vi "ScanDelay_FTIR_GetSpectrum_Aligning_Testing.vi"(0 "Cancel? External":refnum<vi>, 1 "% averaged (external)":refnum<vi>, 2 "Binned interferogram (external)":refnum<vi>, 3 "Python refnum in":refnum<k35>, 5 "Refresh alignment":bool=TRUE, 7 "Acquisition cycle (external)":refnum<vi>, 9 "Delay calibration\n          factor":dbl=2.403, 10 "Python error in":errorcluster, 11 "Subtract\ndelay (ps)":dbl, 12 "Acquisitions per interferogram":i32=20, 13 "Time per\nacquisition (s)":dbl=0.31, 14 "Sampling rate":dbl=250000.0, 15 "Extract envelope":bool=TRUE) -> (4 "Output spectrum":dbl[][](array[numeric]), 6 "Python error out":errorcluster)   [LabVIEW 2021]
uses:
  Control_GetSpectrum_Aligning.ctl
  <vilib>/DAQmx/read.llb/DAQmx Read (Analog 2D DBL NChan NSamp).vi
  <vilib>/DAQmx/miscellaneous.llb/DAQmx Fill In Error Info.vi
panel:
  out "Time per\nloop1 (ms)":dbl=333.0
  out "DAQmx error":errorcluster={"status"=FALSE, "code"=200012, "source"="DAQmx Control Task.vi:3900001"}
  out "Time per\nloop2 (ms)":dbl
  in  "Save interferograms\n(interferograms.txt)":bool
  in  "Alignment order":i32=1
  out "Own python session":bool=TRUE
  out "Refnum errors":errorcluster={"status"=TRUE, "code"=1055, "source"="Property Node in ScanDelay_FTIR_GetSpectrum_Aligning_Testing.vi"}
  out "Spectrum (amplitude)":cluster{dbl[], dbl[]}[](graph)
  out "Spectrum (phase)":cluster{dbl[], dbl[]}(graph)
  out "Interferogram (aligned)":cluster{dbl, dbl}[](graph)
  out "Acquisition cycle":dbl[][](graph)
  in  "Halt acquisition":bool
  out "Python module path":path=path "C:/Users/mnopl/Desktop/Software/LabVIEW/ScanDelay/scandelay.py"
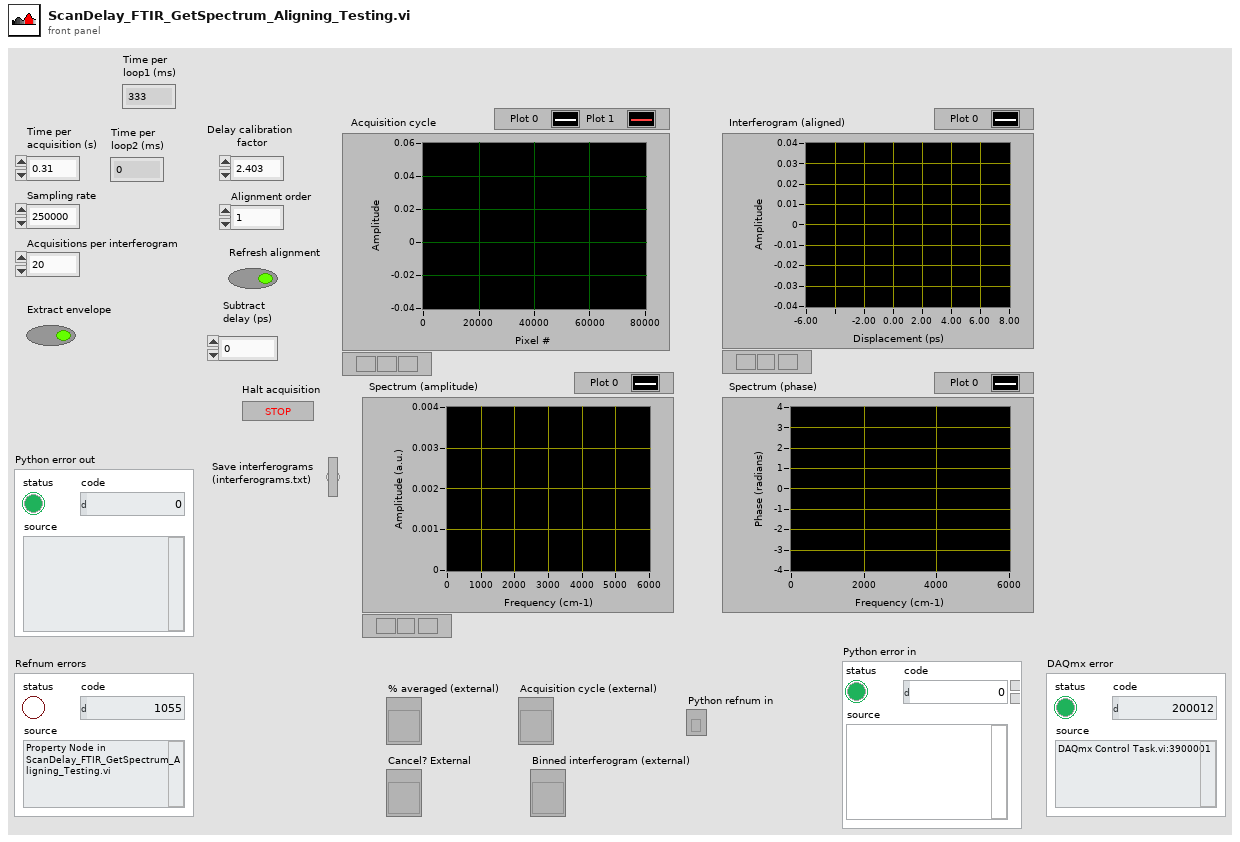
[diagram p1: front panel]
types:
  T1 = typedef "Control_GetSpectrum_Aligning.ctl" = enum16{"Acquire Interferograms", "Prepare DAQ task", "Align Interferograms", "Compute Spectrum", "Done"}
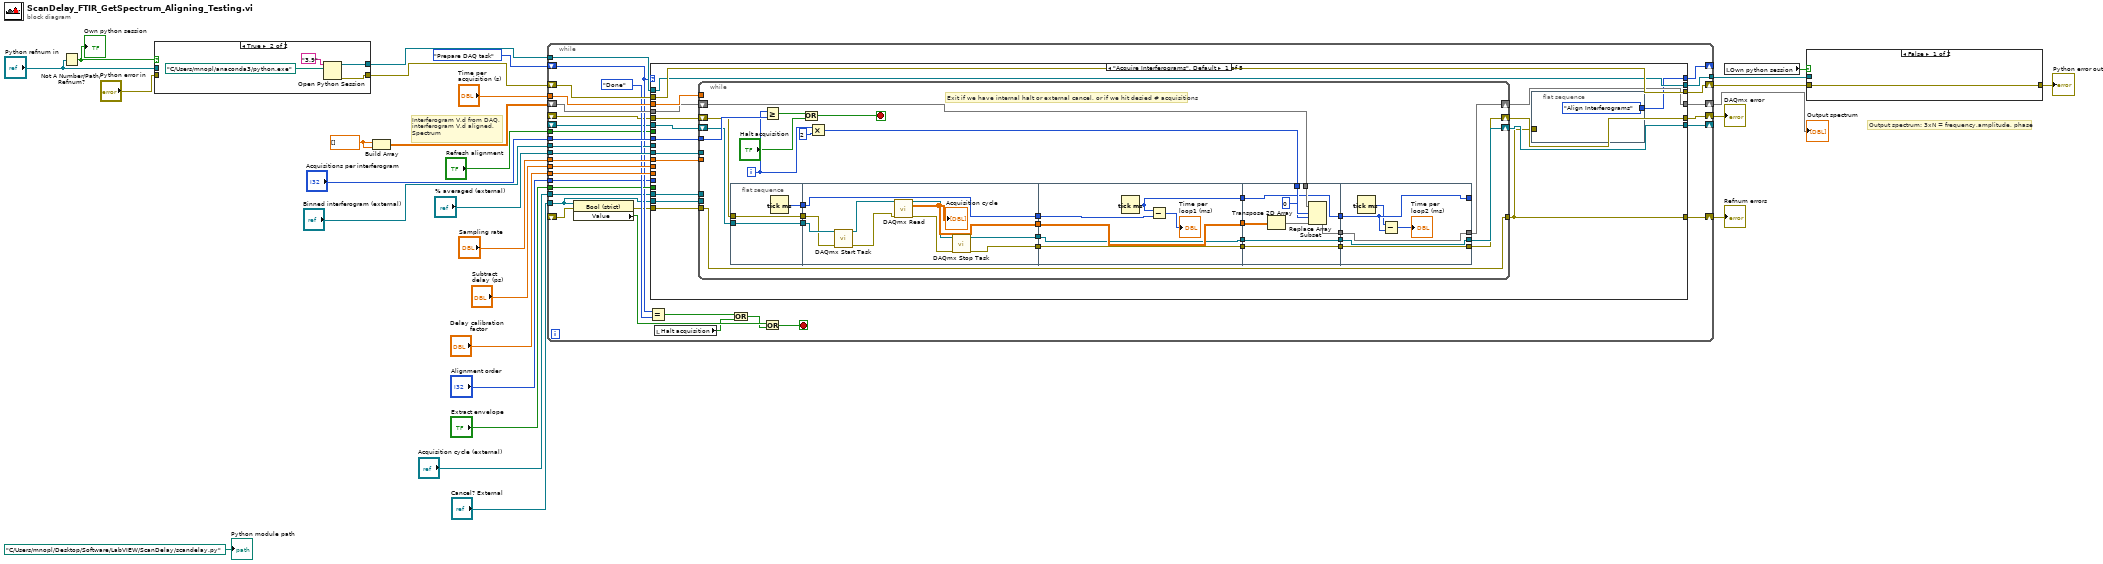
[diagram p0: block diagram]
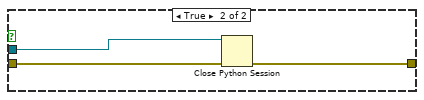
[diagram p2: hidden frame]
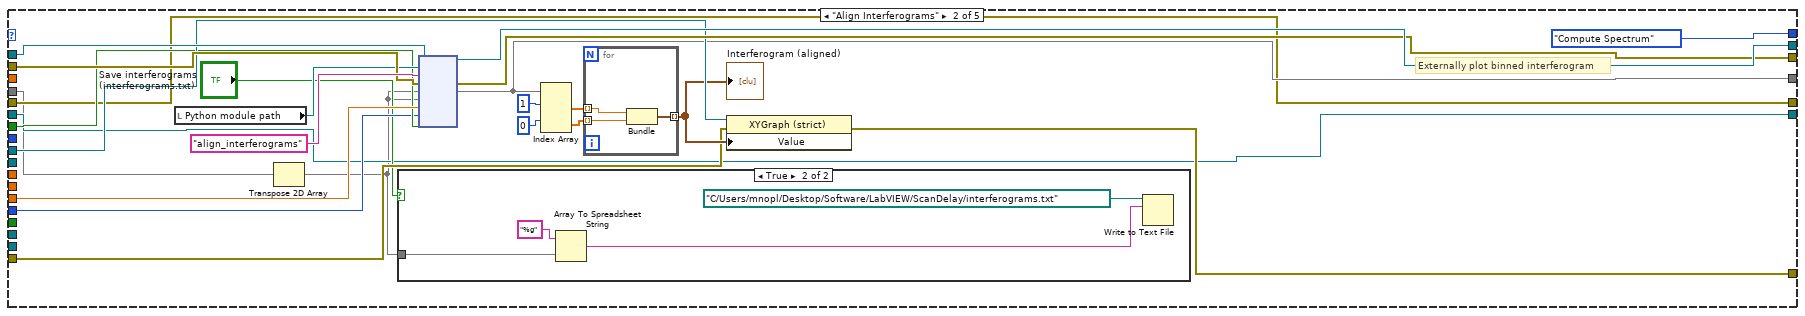
[diagram p4: hidden frame]
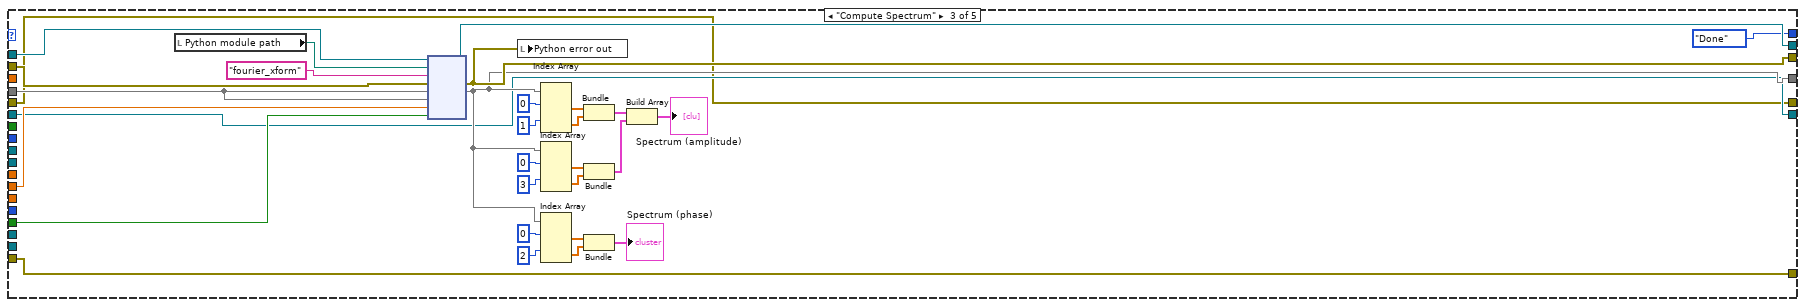
[diagram p6: hidden frame]
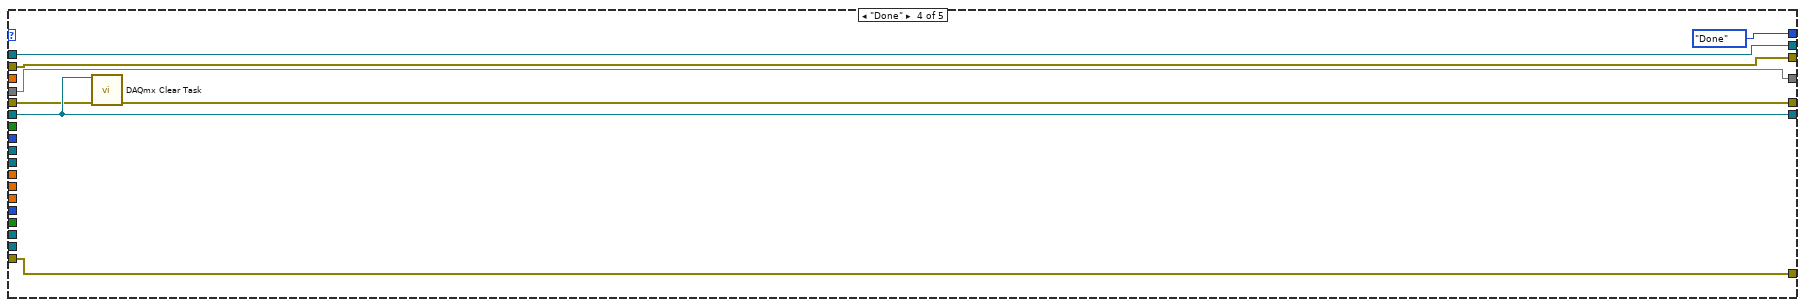
[diagram p7: hidden frame]
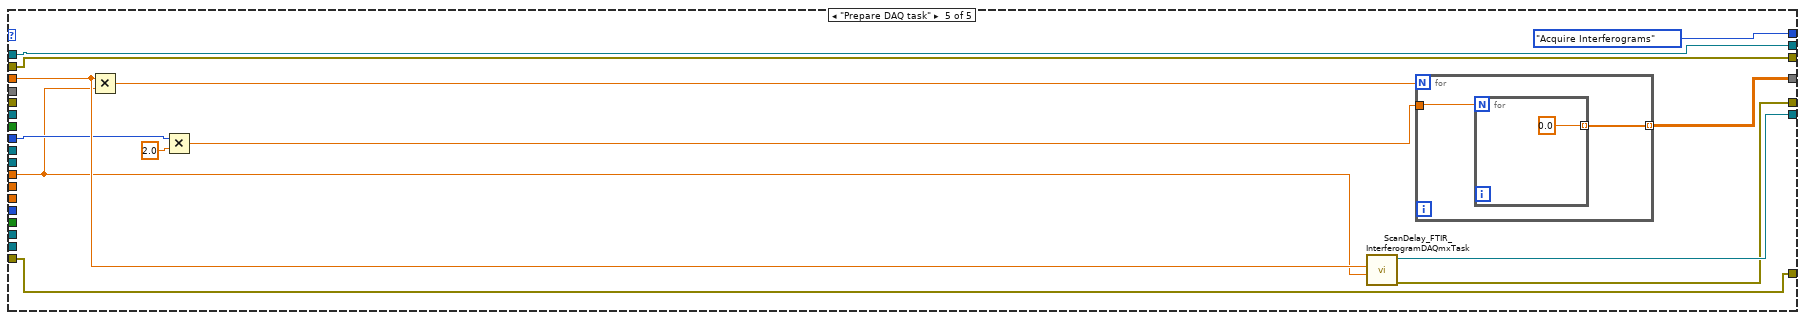
[diagram p8: hidden frame]
diagram:
  w17 = dbl[] []
  # "Output spectrum: 3xN = frequency,amplitude, phase"
  # "Interferogram V,d from DAQ,\ninterferogram V,d aligned,\nSpectrum"
  n1 = Not A Number/Path/Refnum?(number/path/refnum="Python refnum in") -> (NaN/Path/Refnum?=w7:bool)
  "Own python session" <- w7
  n2 = case shown="True" w7 {
    tunnel: [w30 w32] -> w11
    tunnel: [w29 w31] -> w10
    tunnel: "Python refnum in" -> [w30 _]
    tunnel: "Python error in" -> [w29 _]
    frame False {
    }
    frame True {
      n3 = Open Python Session(python version="3.9", python path=path "C:/Users/mnopl/anaconda3/python.exe") -> (session out=w32:refnum<k35>, error out=w31:errorcluster)  [unwired: 1 in]
    }
  }
  n4 = Build Array(w17, w17) -> (w4:dbl[][])
  n5 = while {
    shift-right: [w49] -> w16
    shift-left: w4 -> [w67]
    tunnel: w11 -> [w66]
    tunnel: "Acquisition cycle (external)" -> [w39]
    tunnel: "Sampling rate" -> [w64]
    tunnel: "Time per\nacquisition (s)" -> [w63]
    tunnel: "Delay calibration\n          factor" -> [w62]
    tunnel: "% averaged (external)" -> [w61]
    tunnel: "Cancel? External" -> [w42]
    tunnel: "Acquisitions per interferogram" -> [w60]
    shift-right: [w59] -> _
    shift-left: Control_GetSpectrum_Aligning."Prepare DAQ task" -> [w50]
    tunnel: "Subtract\ndelay (ps)" -> [w58]
    tunnel: [w55] -> w18
    shift-right: [w54] -> w15
    shift-left: w10 -> [w65]
    tunnel: "Extract envelope" -> [w53]
    shift-right: [w52] -> w13
    shift-left: _ -> [w40]
    tunnel: "Binned interferogram (external)" -> [w51]
    tunnel: "Refresh alignment" -> [w48]
    tunnel: "Alignment order" -> [w47]
    shift-right: [w37] -> w1
    shift-left: _ -> [w35]
    shift-right: [w38] -> _
    shift-left: _ -> [w36]
    stop <- w44 stop-if-true
    n6 = property on="Property Node" class="Bool (strict)"(reference=w42, error in=w40) -> (error out=w41:errorcluster, "Value"=w46:bool)  [unwired: 1 out]
    n7 = Equal?(x=w50, y=Control_GetSpectrum_Aligning."Done") -> (x = y?=w56:bool)
    n8 = case shown="\"Acquire Interferograms\", Default" w50 {
      tunnel: w67 -> [w70 w150 w208 w214 _]
      tunnel: w66 -> [w71 w171 w207 w216 w226]
      tunnel: w65 -> [w79 w170 w204 w217 w225]
      tunnel: w39 -> [w84 _ _ _ _]
      tunnel: w64 -> [w83 _ _ _ w220]
      tunnel: w63 -> [w82 _ _ _ w224]
      tunnel: w62 -> [_ w158 _ _ _]
      tunnel: w61 -> [w81 _ _ _ _]
      tunnel: w42 -> [w80 _ _ _ _]
      tunnel: w60 -> [w77 _ _ _ w221]
      tunnel: [w71 w169 w206 w216 w226] -> w55
      tunnel: [w69 Control_GetSpectrum_Aligning."Compute Spectrum" Control_GetSpectrum_Aligning."Done" Control_GetSpectrum_Aligning."Done" Control_GetSpectrum_Aligning."Acquire Interferograms"] -> w59
      tunnel: w58 -> [_ _ w203 _ _]
      tunnel: [w79 w165 w184 w217 w225] -> w54
      tunnel: w53 -> [_ _ w193 _ _]
      tunnel: [w68 w163 w182 w213 w228] -> w52
      tunnel: w51 -> [_ w164 _ _ _]
      tunnel: [w78 w157 w183 w214 w223] -> w49
      tunnel: w48 -> [_ w156 _ _ _]
      tunnel: w47 -> [_ w155 _ _ _]
      tunnel: w41 -> [w76 w154 w182 w213 w228]
      tunnel: [w73 w152 w181 w212 w230] -> w38
      tunnel: [w72 w151 w180 w210 w229] -> w37
      tunnel: w36 -> [w75 w152 w181 w212 _]
      tunnel: w35 -> [w74 w151 w180 w211 _]
      frame "Acquire Interferograms", Default {
        n9 = while {
          tunnel: w84 -> [_]
          tunnel: w83 -> [_]
          tunnel: w82 -> [_]
          tunnel: w81 -> [_]
          tunnel: w80 -> [_]
          tunnel: [w109] -> w68
          shift-right: [w101] -> w78
          shift-left: w70 -> [w103]
          tunnel: w77 -> [w113]
          tunnel: w76 -> [w109]
          shift-right: [w105] -> w73
          shift-left: w75 -> [w107]
          shift-right: [w104] -> w72
          shift-left: w74 -> [w106]
          i -> [w112]
          stop <- w114 stop-if-true
          # "Exit if we have internal halt or external cancel, or if we hit desied # acquisitions"
          n10 = flat-sequence {
            tunnel: w106 -> [w116]
            tunnel: w107 -> [w117]
            tunnel: [w117] -> w96
            tunnel: [w116] -> w95
            tunnel: [w115] -> w94
            tunnel: [w127] -> w93
            tunnel: [w122] -> w91
            tunnel: [w124] -> w90
            tunnel: [w123] -> w88
            tunnel: w96 -> [w119]
            tunnel: w95 -> [w118]
            tunnel: w94 -> [w122]
            tunnel: w93 -> [w133]
            tunnel: [w133] -> w92
            tunnel: w91 -> [w132]
            tunnel: w90 -> [w131]
            tunnel: [w131] -> w89
            tunnel: w88 -> [w130]
            tunnel: [w130] -> w87
            tunnel: [w128] -> w86
            tunnel: w92 -> [w140]
            tunnel: w89 -> [w142]
            tunnel: w87 -> [w141]
            tunnel: w103 -> [w139]
            tunnel: w102 -> [w137]
            tunnel: [w134] -> w100
            tunnel: [w142] -> w99
            tunnel: [w141] -> w98
            tunnel: [w136] -> w97
            tunnel: w86 -> [w134]
            tunnel: [w146] -> w101
            tunnel: [w147] -> w104
            tunnel: [w148] -> w105
            tunnel: [w145] -> _
            tunnel: w100 -> [w145]
            tunnel: w99 -> [w148]
            tunnel: w98 -> [w147]
            tunnel: w97 -> [w146]
            frame #0 {
              n11 = Tick Count (ms)() -> (millisecond timer value=w115:u32)
            }
            frame #1 {
              n12 = call <vilib>:"DAQmx Start Task.vi"("task/channels in"=w119, "error in"=w118) -> ("task out"=w121:refnum<k21>, "error out"=w120:errorcluster)  [unwired: 12 in]
              n13 = call-poly <vilib>:"DAQmx Read.vi"("task/channels in"=w121, "error in"=w120) -> ("task out"=w126:refnum<k21>, "data"=w127:dbl[][], "error out"=w125:errorcluster)  [unwired: 11 in]
              "Acquisition cycle" <- w127
              n14 = call <vilib>:"DAQmx Stop Task.vi"("task/channels in"=w126, "error in"=w125) -> ("task out"=w124:refnum<k21>, "error out"=w123:errorcluster)  [unwired: 12 in]
            }
            frame #2 {
              n15 = Tick Count (ms)() -> (millisecond timer value=w128:u32)
              n16 = Subtract(x=w128, y=w132) -> (x-y=→"Time per\nloop1 (ms)":u32)
            }
            frame #3 {
              n17 = Transpose 2D Array(2D array=w140) -> (transposed array=w135:dbl[][])
              n18 = Replace Array Subset(array=w139, new element=w135, index (row)=0, index (col)=w137) -> (w136:dbl[][])
            }
            frame #4 {
              n19 = Tick Count (ms)() -> (millisecond timer value=w144:u32)
              n20 = Subtract(x=w144, y=w145) -> (x-y=→"Time per\nloop2 (ms)":u32)
            }
          }
          n21 = Greater Or Equal?(x=w112, y=w113) -> (x >= y?=w110:bool)
          n22 = Or(x=w110, y="Halt acquisition") -> (x .or. y?=w114:bool)
          n23 = Multiply(x=w112, y=2) -> (x*y=w102:i32)
        }
        n24 = flat-sequence {
          tunnel: [Control_GetSpectrum_Aligning."Align Interferograms"] -> w69
          tunnel: w68 -> [_]
          frame #0 {
          }
        }
      }
      frame "Align Interferograms" {
        # "Externally plot binned interferogram"
        n25 = local read "Python module path"() -> (w168:path)
        n26 = Transpose 2D Array(2D array=w150) -> (transposed array=w149:dbl[][])
        n27 = case shown="True" "Save interferograms\n(interferograms.txt)" {
          tunnel: w149 -> [_ w174]
          frame False {
          }
          frame True {
            n28 = Array To Spreadsheet String(array=w174, 3:"%g") -> (spreadsheet string=w176:string)  [unwired: 1 in]
            n29 = Write to Text File(file (use dialog)=path "C:/Users/mnopl/Desktop/Software/LabVIEW/ScanDelay/interferograms.txt", text=w176) -> ()  [unwired: 2 in, 3 out]
          }
        }
        n30 = node(w171, w168, "align_interferograms", w170, w149, w149, w158, w155, w156) -> (w169:refnum<k35>, w165:errorcluster, w157:dbl[][])  [unwired: 4 in, 2 out]
        n31 = Index Array(array=w157, index (row) #1=1, index (row) #2=0) -> (element #1=w161:dbl[], element #2=w162:dbl[])  [unwired: 2 in]
        n32 = for {
          tunnel: w162 -> [w178] mode=indexing
          tunnel: w161 -> [w179] mode=indexing
          tunnel: [w177] -> w160 mode=indexing
          n33 = Bundle(w179, w178) -> (w177:cluster{dbl, dbl})  [unwired: 1 in]
        }
        "Interferogram (aligned)" <- w160
        n34 = property on="Property Node" class="XYGraph (strict)"(reference=w164, error in=w154, "Value"=w160) -> (error out=w163:errorcluster)  [unwired: 1 out]
      }
      frame "Compute Spectrum" {
        n35 = local read "Python module path"() -> (w205:path)
        n36 = node(w207, w205, "fourier_xform", w204, w208, w208, w203, w193) -> (w206:refnum<k35>, w184:errorcluster, w183:dbl[][])  [unwired: 3 in, 2 out]
        n37 = local write "Python error out"(w184) -> ()
        n38 = Index Array(array=w183, index (row) #1=0, index (row) #2=1) -> (element #1=w199:dbl[], element #2=w198:dbl[])  [unwired: 2 in]
        n39 = Index Array(array=w183, index (row) #1=0, index (row) #2=3) -> (element #1=w194:dbl[], element #2=w195:dbl[])  [unwired: 2 in]
        n40 = Index Array(array=w183, index (row) #1=0, index (row) #2=2) -> (element #1=w189:dbl[], element #2=w190:dbl[])  [unwired: 2 in]
        n41 = Bundle(w199, w198) -> (w187:cluster{dbl[], dbl[]})  [unwired: 1 in]
        n42 = Bundle(w194, w195) -> (w186:cluster{dbl[], dbl[]})  [unwired: 1 in]
        n43 = Bundle(w189, w190) -> (→"Spectrum (phase)":cluster{dbl[], dbl[]})  [unwired: 1 in]
        n44 = Build Array(w187, w186) -> (→"Spectrum (amplitude)":cluster{dbl[], dbl[]}[])
      }
      frame "Done" {
        n45 = call <vilib>:"DAQmx Clear Task.vi"("task in"=w212, "error in"=w211) -> ("error out"=w210:errorcluster)  [unwired: 13 in]
      }
      frame "Prepare DAQ task" {
        n46 = Multiply(x=w224, y=w220) -> (x*y=w219:dbl)
        n47 = Multiply(x=w221, y=2.0) -> (x*y=w218:dbl)
        n48 = call "ScanDelay_FTIR_InterferogramDAQmxTask.vi"("Sampling rate"=w220, "Time per acquisiton (s)"=w224) -> ("error out"=w229:errorcluster, "Refnum out"=w230:refnum<k21>)  [unwired: 8 in]
        n49 = for {
          N: w219 -> [_]
          tunnel: [w232] -> w223 mode=indexing
          tunnel: w218 -> [w231]
          n50 = for {
            N: w231 -> [_]
            tunnel: [0.0] -> w232 mode=indexing
          }
        }
      }
    }
    n51 = local read "Halt acquisition"() -> (w43:bool)
    n52 = Or(x=w56, y=w43) -> (x .or. y?=w45:bool)
    n53 = Or(x=w46, y=w45) -> (x .or. y?=w44:bool)
  }
  "Output spectrum" <- w16
  "Refnum errors" <- w13
  "DAQmx error" <- w1
  n54 = local read "Own python session"() -> (w6:bool)
  n55 = case shown="False" w6 {
    tunnel: [w234 w237] -> w19
    tunnel: w18 -> [_ w236]
    tunnel: w15 -> [w234 w235]
    frame False {
    }
    frame True {
      n56 = Close Python Session(session in=w236, error in=w235) -> (11:w237:errorcluster)
    }
  }
  "Python error out" <- w19
  "Python module path" <- path "C:/Users/mnopl/Desktop/Software/LabVIEW/ScanDelay/scandelay.py"
